vi "InitBrooks.vi"(8 "error in":errorcluster, 9 "TAG":string="27294009", 10 "Baud":i32=19200, 11 "COM":i32=9) -> (0 "error out":errorcluster, 1 "IDS":u8 format="%.0x", 2 "IDL":u8 format="%.0x", 3 "IDM":u8 format="%.0x", 5 "IDH":u8 format="%.0x")   [LabVIEW 2012]
uses:
  S Protocol/BrooksDLL.dll
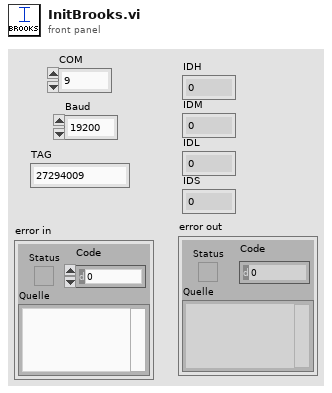
[diagram p1: front panel]
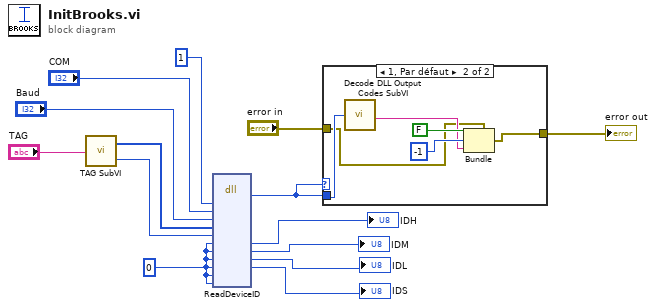
[diagram p0: block diagram]
diagram:
  w9 = u8 0
  n1 = call "TAG SubVI.vi"("TAG String"="TAG") -> ("TAG"=w11:u8[], "Length"=w10:i32)
  n2 = dll-call lib="C:/Users/Sylvain/Desktop/TopPerm_20150127/drivers/Brooks/S Protocol/BrooksDLL.dll" fn="ReadDeviceID"("DropType"=u8 1, "COM"="COM", "Baud"="Baud", "TAG"=w11, "Length"=w10, "IDH"=w9, "IDM"=w9, "IDL"=w9, "IDS"=w9, "S1"=w9, "S2"=w9) -> (w3:i32, "IDH"=→"IDH":u8, "IDM"=→"IDM":u8, "IDL"=→"IDL":u8, "IDS"=→"IDS":u8)  [unwired: 10 in, 2 out]
  n3 = case shown="1, Par défaut" w3 {
    tunnel: w3 -> [_ w21]
    tunnel: "error in" -> [w15 w17]
    tunnel: [w15 w16] -> w1
    frame 0 {
    }
    frame 1, Default {
      n4 = call "Decode DLL Output Codes SubVI.vi"("Numeric"=w21) -> ("Function Output Comment"=w18:string)
      n5 = Bundle(cluster=w17, "status"=FALSE, "code"=-1, "source"=w18) -> (w16:errorcluster)
    }
  }
  "error out" <- w1
